vi "execute_protocol_topLvl.vi"(5 "which manipulator":T1(ring), 7 "Slide Refnum":refnum<vi>, 8 "error in":errorcluster, 10 "protocol array":dbl[][](array[numeric])=[[10.0, -200.0], [60.0, 1000.0], [10.0, -200.0], [60.0, 1000.0], [10.0, -200.0], [60.0, 1000.0], [10.0, -200.0], [60.0, 1000.0], [10.0, -200.0], [60.0, 1000.0], [10.0, -200.0], [60.0, 1000.0], [10.0, -200.0], [60.0, 1000.0], [10.0, -200.0], [60.0, 1000.0], [10.0, -200.0], [60.0, 1000.0], [10.0, -200.0], [60.0, 1000.0]], 11 "Pressure box control in":T2={"Pressure box COM"="", "pressure box type"=enum."Neuromatics", "High pos pressure (mBar)"=200.0, "Low pos pressure (mBar)"=80.0, "Vacuum pressure (mBar)"=-40.0, "calibration"=enum."PA_vacPump"}) -> (0 "error out":errorcluster, 3 "Pressure box control out":T2={"Pressure box COM"="", "pressure box type"=enum."Neuromatics", "High pos pressure (mBar)"=200.0, "Low pos pressure (mBar)"=80.0, "Vacuum pressure (mBar)"=-40.0, "calibration"=enum."PA_vacPump"})   [LabVIEW 2015]
uses:
  controls/pressure_box_type.ctl
  controls/pressure_box_control.ctl
panel:
  out "step #":i32
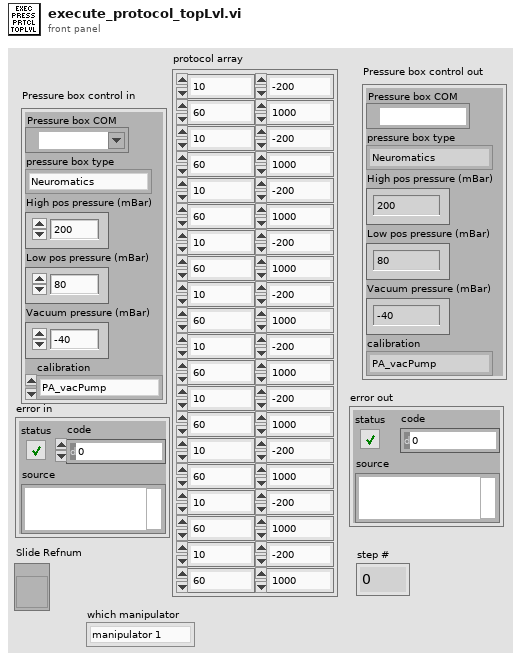
[diagram p1: front panel]
types:
  T1 = enum16{"manipulator 1", "manipulator 2", "manipulator 3", "manipulator 4"}
  T2 = typedef "pressure_box_control.ctl" = cluster{"Pressure box COM":refnum<visa-resource-name>, "pressure box type":T3, "High pos pressure (mBar)":dbl, "Low pos pressure (mBar)":dbl, "Vacuum pressure (mBar)":dbl, "calibration":enum16{"PA_vacPump", "PA_venturi", "Neuromatics", "ilyaRig", "mightenRig"}}
  T3 = typedef "pressure_box_type.ctl" = enum16{"Neuromatics", "ProportionAir", "Demo box", "N-ProportionAir"}
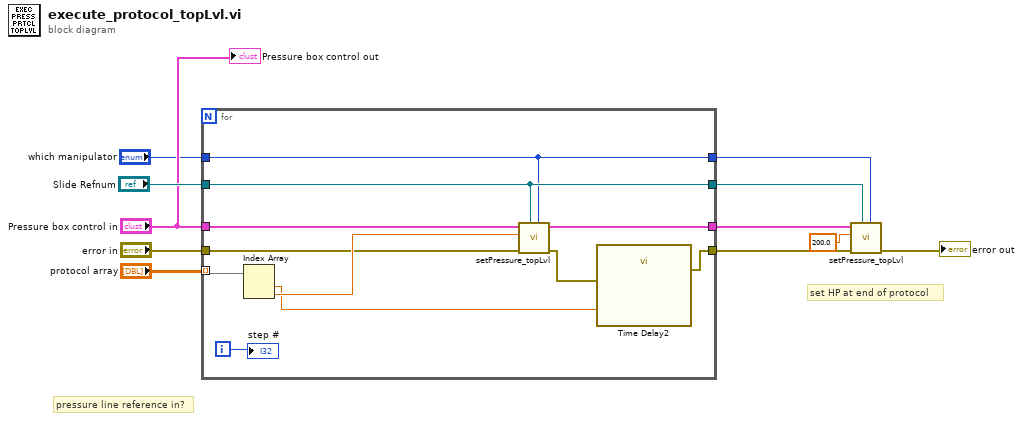
[diagram p0: block diagram]
diagram:
  # "pressure line reference in?"
  # "set HP at end of protocol"
  n1 = for {
    tunnel: "protocol array" -> [w22] mode=indexing
    tunnel: "error in" -> [w20]
    tunnel: [w19] -> w9
    tunnel: [w15] -> w4
    tunnel: "Slide Refnum" -> [w14]
    tunnel: [w14] -> w5
    tunnel: "Pressure box control in" -> [w13]
    tunnel: "which manipulator" -> [w12]
    tunnel: [w12] -> w1
    i -> [w18]
    n2 = Index Array(array=w22) -> (element #1=w17:dbl, element #2=w21:dbl)  [unwired: 2 in]
    n3 = call "setPressure_topLvl.vi"("which manipulator"=w12, "Slide Refnum"=w14, "error in"=w20, "set pressure (mBar)"=w21, "Pressure box control in"=w13) -> ("error out"=w16:errorcluster, "Pressure box control out"=w15:T2)  [unwired: 5 in]
    n4 = call "Time Delay2"("error in (no error)"=w16, "Delay Time (s)"=w17) -> ("error out"=w19:errorcluster)  [unwired: 9 in]
    "step #" <- w18
  }
  n5 = call "setPressure_topLvl.vi"("which manipulator"=w1, "Slide Refnum"=w5, "error in"=w9, "set pressure (mBar)"=200.0 ("pressure set (mBar)"), "Pressure box control in"=w4) -> ("error out"=→"error out":errorcluster)  [unwired: 5 in, 1 out]
  "Pressure box control out" <- "Pressure box control in"
